vi "Aircraft 1 Extra Data .vi"(7 "Method":enum16{"Get", "Set"}(ring), 11 "Extra Data In":T1) -> (3 "Extra Data Out":T1)   [LabVIEW 2014]
uses:
  Controls/Aircraft Extra Data.ctl
  MAVLink/Controls/MAVLink Optical Flow.ctl
  MAVLink/Controls/MAVLink EKF Status Report.ctl
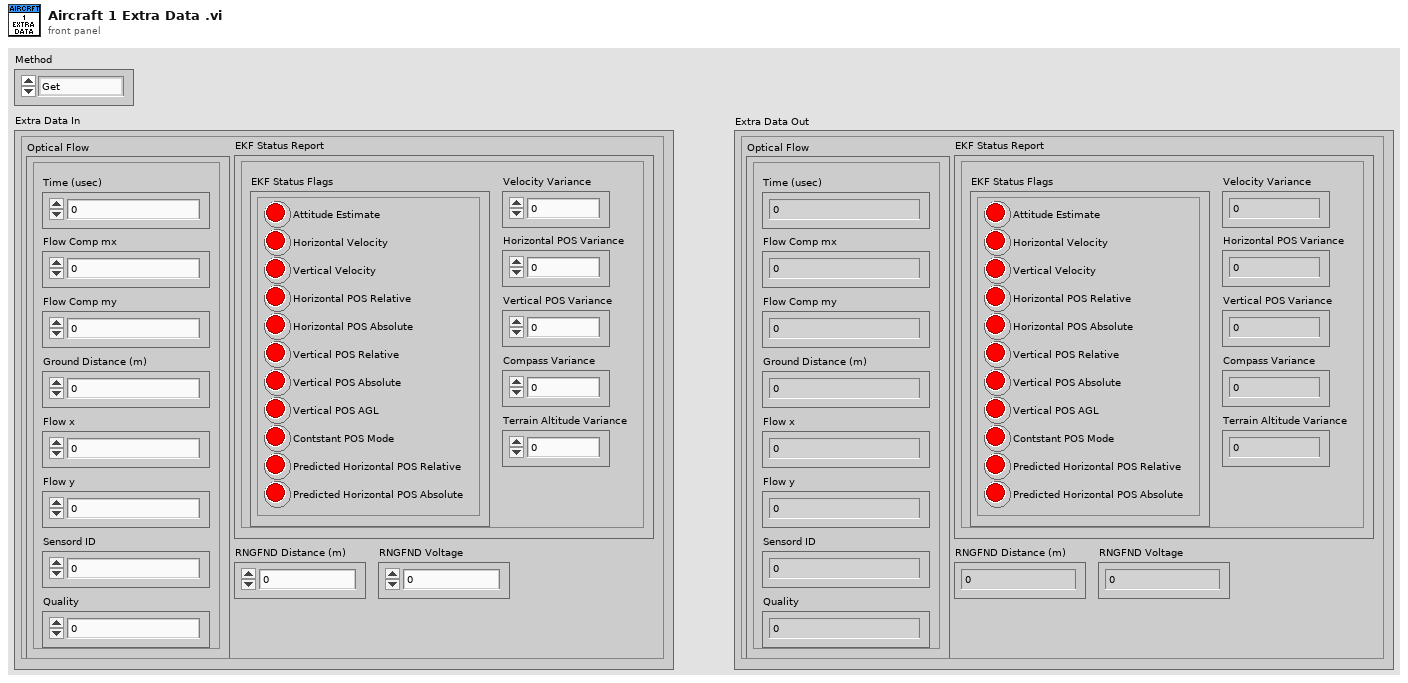
[diagram p1: front panel]
types:
  T1 = typedef "Aircraft Extra Data.ctl" = cluster{"Optical Flow":T2, "RNGFND Distance (m)":sgl, "RNGFND Voltage":sgl, "EKF Status Report":T3}
  T2 = typedef "MAVLink Optical Flow.ctl" = cluster{"Time (usec)":u64, "Flow Comp mx":sgl, "Flow Comp my":sgl, "Ground Distance (m)":sgl, "Flow x":i16, "Flow y":i16, "Sensord ID":u8, "Quality":u8}
  T3 = typedef "MAVLink EKF Status Report.ctl" = cluster{"EKF Status Flags":cluster{"Attitude Estimate":bool, "Horizontal Velocity":bool, "Vertical Velocity":bool, "Horizontal POS Relative":bool, "Horizontal POS Absolute":bool, "Vertical POS Relative":bool, "Vertical POS Absolute":bool, "Vertical POS AGL":bool, "Contstant POS Mode":bool, "Predicted Horizontal POS Relative":bool, "Predicted Horizontal POS Absolute":bool}, "Velocity Variance":sgl, "Horizontal POS Variance":sgl, "Vertical POS Variance":sgl, "Compass Variance":sgl, "Terrain Altitude Variance":sgl}
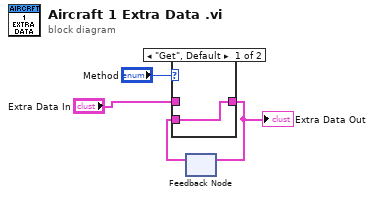
[diagram p0: block diagram]
diagram:
  n1 = feedback #1() -> (w3:T1)  [unwired: 1 in]
  n2 = case shown="\"Get\", Default" "Method" {
    tunnel: "Extra Data In" -> [_ w6]
    tunnel: [w5 w6] -> w2
    tunnel: w3 -> [w5 _]
    frame "Get", Default {
    }
    frame "Set" {
    }
  }
  "Extra Data Out" <- w2
  n3 = feedback-in #1(w2) -> ()
